vi "main2.vi"() -> ()   [LabVIEW 2011]
uses:
  genericVehicle/vehicleGeneric.lvclass
  car/car.lvclass
  bike/bike.lvclass
panel:
  out "numberOfWheels":dbl
  out "Array":dbl[](array[numeric])
  in  "Cluster":T1
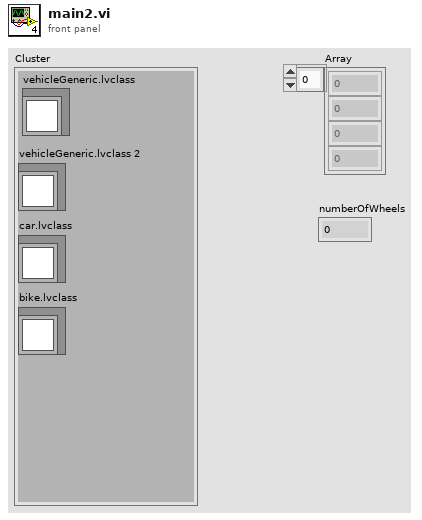
[diagram p1: front panel]
types:
  T1 = cluster{"vehicleGeneric.lvclass":refnum<class "vehicleGeneric.lvclass">, "vehicleGeneric.lvclass 2":refnum<class "vehicleGeneric.lvclass">, "car.lvclass":refnum<class "car.lvclass">, "bike.lvclass":refnum<class "bike.lvclass">}
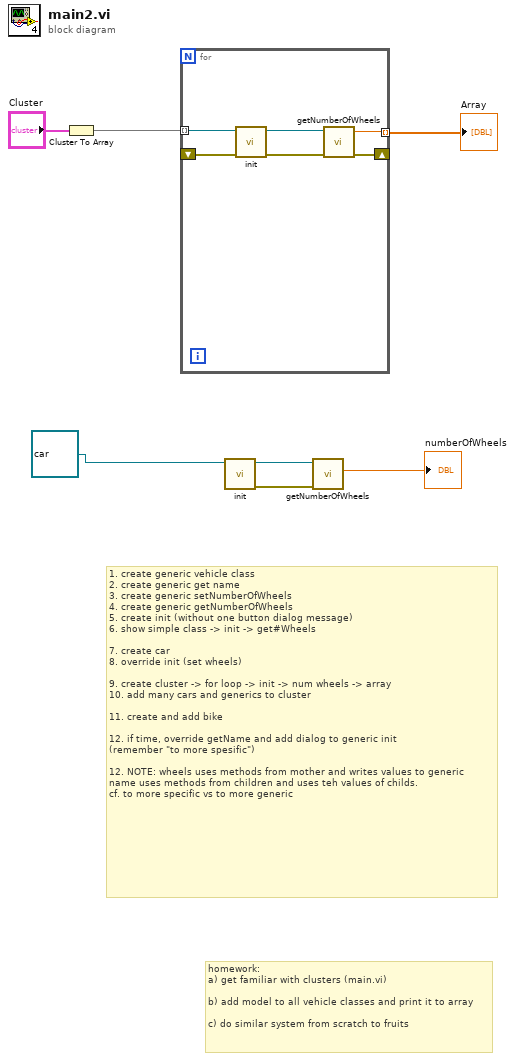
[diagram p0: block diagram]
diagram:
  # "homework: \na) get familiar with clusters (main.vi)\n\nb) add model to all vehicle classes and print it to array\n\nc) do similar system from scratch to fruits"
  # "1. create generic vehicle class\n2. create generic get name\n3. create generic setNumberOfWheels\n4. create generic getNumberOfWheels\n5. create init (without one button dialog message)\n6. show simple class -> init -> get#Wheels\n\n7. create car\n8. override init (set wheels)\n\n9. create cluster -> for loop -> init -> num wheels -> array\n10. add many cars and generics to cluster\n\n11. create and add bike\n\n12. if time, override getName and add dialog to generic init\n(remember \"to more spesific\")\n \n12. NOTE: wheels uses methods from mother and writes values to generic\nname uses methods from children and uses teh values of childs.\ncf. to more specific vs to more generic"
  n1 = Cluster To Array(cluster="Cluster") -> (array=w6:refnum<class "vehicleGeneric.lvclass">[])
  n2 = for {
    tunnel: w6 -> [w11] mode=indexing
    tunnel: [w13] -> w5 mode=indexing
    shift-right: [w12] -> _
    shift-left: _ -> [w10]
    n3 = call-dynamic "init.vi"("error in (no error)"=w10, "vehicleGeneric in"=w11) -> ("error out"=w9:errorcluster, "vehicleGeneric out"=w8:refnum<class "vehicleGeneric.lvclass">)  [unwired: 8 in]
    n4 = call-dynamic "getNumberOfWheels.vi"("error in (no error)"=w9, "vehicle in"=w8) -> ("error out"=w12:errorcluster, "numberOfWheels"=w13:dbl)  [unwired: 7 in, 1 out]
  }
  "Array" <- w5
  n5 = call-dynamic "init.vi"("car in"=refnum<class "car.lvclass"> refnum ("car.lvclass")) -> ("error out"=w3:errorcluster, "car out"=w4:refnum<class "car.lvclass">)  [unwired: 9 in]
  n6 = call-dynamic "getNumberOfWheels.vi"("error in (no error)"=w3, "vehicle in"=w4) -> ("numberOfWheels"=→"numberOfWheels":dbl)  [unwired: 7 in, 2 out]
